vi "AI Waveform Scan Stub.vi"(0 "stop":bool, 2 "Point Number":i32, 3 "Board Number":i16, 4 "Numeric":dbl, 5 "input limits (no change)":T1(array[cluster]), 6 "Number to Average":i32, 7 "channels (0)":string[](array[string])) -> (1 "scaled data":sgl[][](array[numeric]))   [LabVIEW 2020]
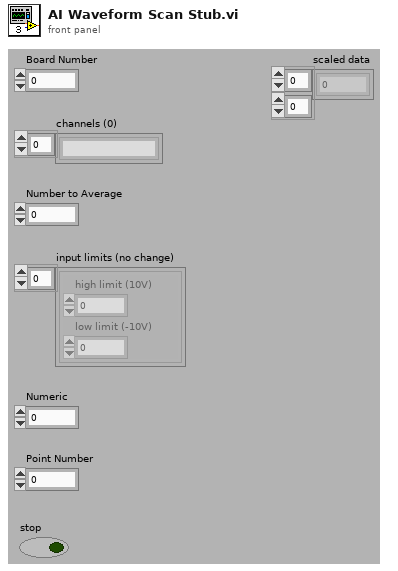
[diagram p1: front panel]
types:
  T1 = cluster{"high limit (10V)":sgl, "low limit (-10V)":sgl}[]
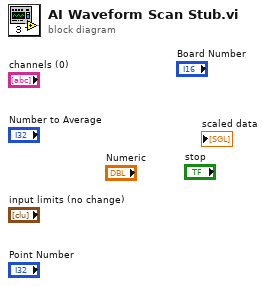
[diagram p0: block diagram]
diagram:
